vi "DHE_SetFPAname.vi"(1 "Path":path=path "", 2 "DHE_FPAname":string) -> ()   [LabVIEW 2016]
uses:
  private/vis/DHE_GBLDriverVariables.vi
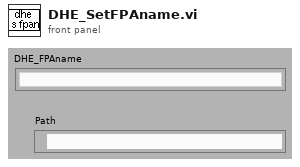
[diagram p1: front panel]
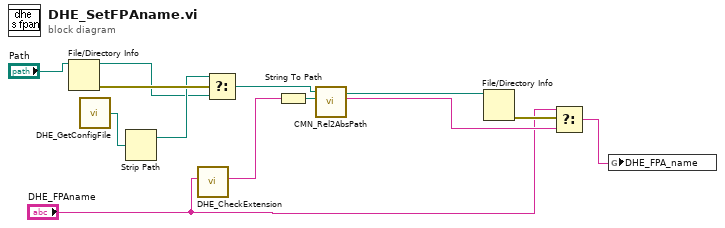
[diagram p0: block diagram]
diagram:
  n1 = File/Directory Info(path="Path") -> (path out=w8:path, error out=w10:errorcluster)  [unwired: 1 in, 5 out]
  n2 = call "DHE_GetConfigFile.vi"() -> ("DHE_ConfigFile"=w12:path)  [unwired: 9 out]
  n3 = Strip Path(path=w12) -> (stripped path=w9:path)  [unwired: 1 out]
  n4 = call "DHE_CheckExtension.vi"("name in"="DHE_FPAname") -> ("name out"=w1:string)  [unwired: 9 out]
  n5 = Select(t=w9, s=w10, f=w8) -> (s? t:f=w5:path)
  n6 = String To Path(string=w1) -> (path=w13:path)
  n7 = call "CMN_Rel2AbsPath.vi"("test path"=w13, "absolute path"=w5) -> ("output path (str)"=w4:string, "output path"=w3:path)  [unwired: 1 in, 7 out]
  n8 = File/Directory Info(path=w3) -> (error out=w7:errorcluster)  [unwired: 1 in, 6 out]
  n9 = Select(t="DHE_FPAname", s=w7, f=w4) -> (s? t:f=w6:string)
  n10 = global write "DHE_GBLDriverVariables.vi" "DHE_FPA_name"(w6) -> ()
